vi "delme2.vi"   [LabVIEW 2020]
uses:
  <vilib>/Utility/miscctls.llb/LVBoundsTypeDef.ctl
panel:
  # "FUCK"
types:
  T1 = typedef "LVBoundsTypeDef.ctl" = cluster{"Width":u32, "Height":u32}
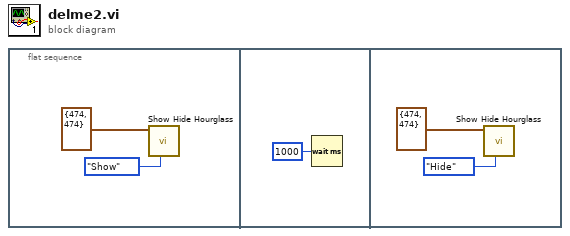
[diagram p0: block diagram]
diagram:
  n1 = flat-sequence {
    frame #0 {
      n2 = call "Show Hide Hourglass.vi"("Action"=enum16{"Hide", "Show"}."Show", "Pic Size"=T1 {"Width"=474, "Height"=474}) -> ()  [unwired: 9 in, 1 out]
    }
    frame #1 {
      n3 = Wait (ms)(milliseconds to wait=u32 1000) -> ()  [unwired: 1 out]
    }
    frame #2 {
      n4 = call "Show Hide Hourglass.vi"("Action"=enum16{"Hide", "Show"}."Hide", "Pic Size"=T1 {"Width"=474, "Height"=474}) -> ()  [unwired: 9 in, 1 out]
    }
  }
